vi "Read Exp sel #.vi"(8 "error in (no error)":errorcluster, 11 "Experiments_group in":refnum<class "Experiments_group.lvclass">) -> (0 "error out":errorcluster, 2 "Exp sel #":i32, 3 "Experiments_group out":refnum<class "Experiments_group.lvclass">)   [LabVIEW 2015, in "Experiments_group.lvclass"]
uses:
  Experiments_group.lvclass
  Experiments_group.lvclass/Experiments_group.ctl
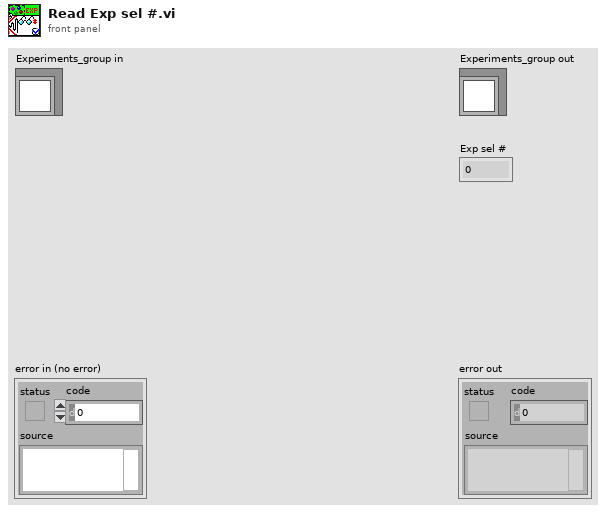
[diagram p1: front panel]
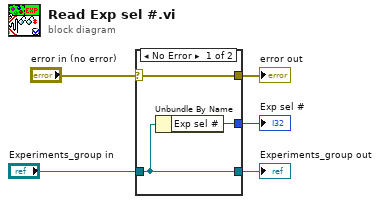
[diagram p0: block diagram]
diagram:
  n1 = case shown="No Error" "error in (no error)" {
    selector: "error in (no error)" -> [w8 w9]
    tunnel: [w8 w9] -> w4
    tunnel: [w7 w10] -> w2
    tunnel: "Experiments_group in" -> [w7 w10]
    tunnel: [w6 _] -> w1
    frame No Error {
      n2 = Unbundle By Name(w7) -> ("Exp sel #"=w6:i32)
    }
    frame Error {
    }
  }
  "error out" <- w4
  "Experiments_group out" <- w2
  "Exp sel #" <- w1
